vi "Delete Link.vi"(8 "Error In":errorcluster, 10 "Remote Path":string, 11 "SFTP In":refnum<class "SFTP.lvclass">) -> (0 "Error Out":errorcluster, 3 "SFTP Out":refnum<class "SFTP.lvclass">)   [LabVIEW 2018, in "Toolkit.lvlib" / "SFTP.lvclass"]
uses:
  SFTP.lvclass
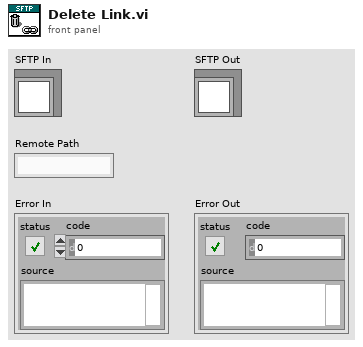
[diagram p1: front panel]
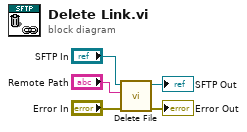
[diagram p0: block diagram]
diagram:
  n1 = call "Delete File.vi"("Error In"="Error In", "Remote Path"="Remote Path", "SFTP In"="SFTP In") -> ("Error Out"=→"Error Out":errorcluster, "SFTP Out"=→"SFTP Out":refnum<class "SFTP.lvclass">)  [unwired: 7 in]
